vi "Add Bookmark Tree Item.vi"(8 "Error In":errorcluster, 9 "Parent Tag":string, 10 "VI Bookmark":T1, 11 "TreeControl In":refnum<vi>) -> (0 "Error Out":errorcluster, 3 "TreeControl Out":refnum<vi>)   [LabVIEW 2017, in "Bookmark Manager.lvlib"]
uses:
  Bookmark Manager.lvlib
  Controls/VI Bookmark.ctl
  Controls/VI Information.ctl
  Controls/Application Information.ctl
  Toolkit VIs/Typedefs/Bookmark Tags.ctl
  Toolkit VIs/Toolkit.lvlib
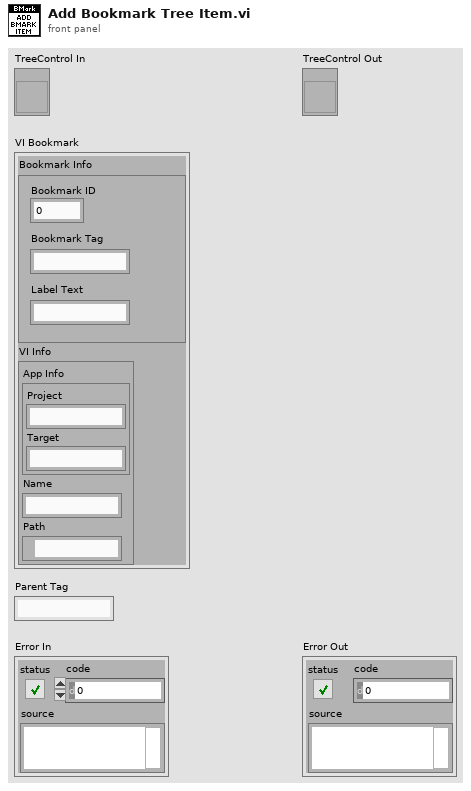
[diagram p1: front panel]
types:
  T1 = typedef "Bookmark Manager.lvlib/VI Bookmark.ctl" = cluster{"Bookmark Info":cluster{"Bookmark ID":u32, "Bookmark Tag":string, "Label Text":string}, "VI Info":T2}
  T2 = typedef "Bookmark Manager.lvlib/VI Information.ctl" = cluster{"App Info":T3, "Name":string, "Path":path}
  T3 = typedef "Bookmark Manager.lvlib/Application Information.ctl" = cluster{"Project":string, "Target":string}
  T4 = typedef "Toolkit.lvlib/Bookmark Tags.ctl" = enum16{"RIP", "Zombie"}
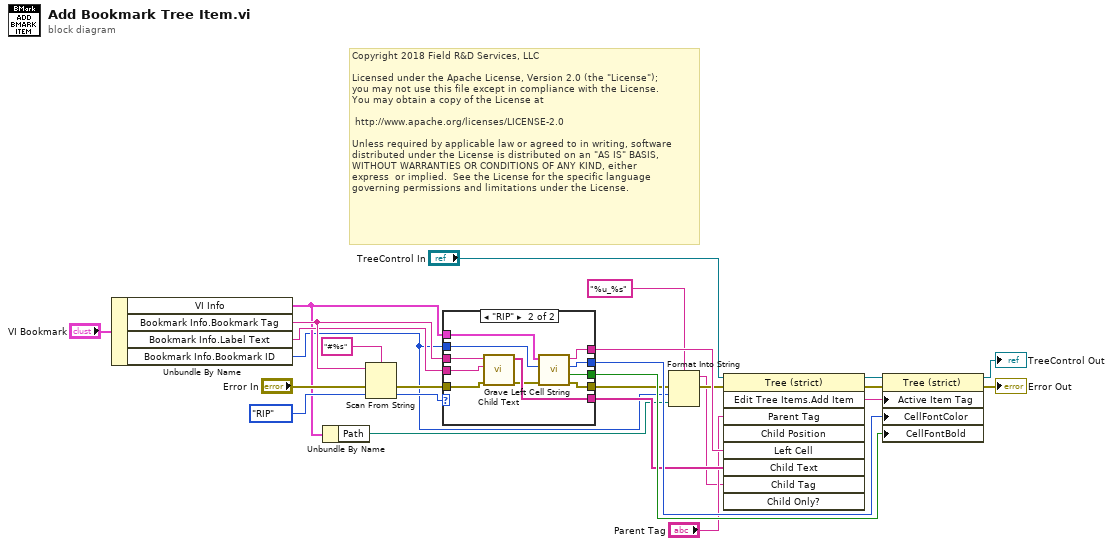
[diagram p0: block diagram]
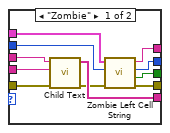
[diagram p2: hidden frame]
diagram:
  # "Copyright 2018 Field R&D Services, LLC\n\nLicensed under the Apache License, Version 2.0 (the \"License\");\nyou may not use this file except in compliance with the License.\nYou may obtain a copy of the License at\n\n\thttp://www.apache.org/licenses/LICENSE-2.0\n\nUnless required by applicable law or agreed to in writing, software\ndistributed under the License is distributed on an \"AS IS\" BASIS,\nWITHOUT WARRANTIES OR CONDITIONS OF ANY KIND, either \nexpress  or implied.  See the License for the specific language \ngoverning permissions and limitations under the License."
  n1 = Unbundle By Name("VI Bookmark") -> ("VI Info"=w6:T2, "Bookmark Info.Bookmark Tag"=w18:string, "Bookmark Info.Label Text"=w10:string, "Bookmark Info.Bookmark ID"=w3:u32)
  n2 = Unbundle By Name(w6) -> ("Path"=w1:path)
  n3 = Scan From String(format string="#%s", input string=w18, error in="Error In", default 1=Bookmark_Tags."RIP" ("Bookmark")) -> (error out=w14:errorcluster, output 1=w16:T4)  [unwired: 1 in, 2 out]
  n4 = case shown="\"RIP\"" w16 {
    tunnel: [w31 w42] -> w23
    tunnel: w10 -> [w36 w47]
    tunnel: [w35 w48] -> w11
    tunnel: w14 -> [w37 w46]
    tunnel: [w30 w41] -> w13
    tunnel: w18 -> [w34 w45]
    tunnel: w3 -> [w32 w44]
    tunnel: [w29 w40] -> w24
    tunnel: [w28 w39] -> w25
    tunnel: w6 -> [w27 w38]
    frame "Zombie" {
      # "Grave"
      n5 = call "Child Text.vi"("Error In"=w37, "Label Text"=w36, "Bookmark Tag"=w34) -> ("Error Out"=w33:errorcluster, "Child Text"=w35:string[])  [unwired: 7 in]
      n6 = call "Zombie Left Cell String.vi"("Error In"=w33, "Bookmark ID"=w32, "VI Info"=w27) -> ("Error Out"=w30:errorcluster, "Bold?"=w28:bool, "Color"=w29:u32, "Text"=w31:string)  [unwired: 5 in]
    }
    frame "RIP" {
      # "Zombie"
      n7 = call "Child Text.vi"("Error In"=w46, "Label Text"=w47, "Bookmark Tag"=w45) -> ("Error Out"=w43:errorcluster, "Child Text"=w48:string[])  [unwired: 7 in]
      n8 = call "Grave Left Cell String.vi"("Error In"=w43, "Bookmark ID"=w44, "VI Info"=w38) -> ("Error Out"=w41:errorcluster, "Bold?"=w39:bool, "Color"=w40:u32, "Text"=w42:string)  [unwired: 5 in]
    }
  }
  n9 = Format Into String(format string="%u_%s", error in=w13, w3, w1) -> (resulting string=w2:string, error out=w5:errorcluster)  [unwired: 1 in]
  n10 = invoke class="Tree (strict)" method="Edit Tree Items.Add Item"(reference="TreeControl In", error in=w5, "Parent Tag"="Parent Tag", "Left Cell"=w23, "Child Text"=w11, "Child Tag"=w2) -> (reference out=w8:refnum<vi>, error out=w20:errorcluster, "Edit Tree Items:Add Item"=w22:string)  [unwired: 3 in, 6 out]
  n11 = property class="Tree (strict)"(reference=w8, error in=w20, "Active Item Tag"=w22, "CellFontColor"=w24, "CellFontBold"=w25) -> (reference out=→"TreeControl Out":refnum<vi>, error out=→"Error Out":errorcluster)
